vi "fetch_image.vi"(8 "error in (no error)":errorcluster, 11 "GenericToplevelComponent in":refnum<class "GenericToplevelComponent.lvclass">) -> (0 "error out":errorcluster, 1 "channels array empty?":bool, 2 "image (channels)":refnum<class "Image.lvclass">[](array[class]), 3 "GenericToplevelComponent out":refnum<class "GenericToplevelComponent.lvclass">, 4 "# elements in queue":i32, 6 "finished?":bool[](array[boolean]))   [LabVIEW 2010, in "GenericToplevelComponent.lvclass"]
uses:
  GenericToplevelComponent.lvclass
  Image/Image/Image.lvclass
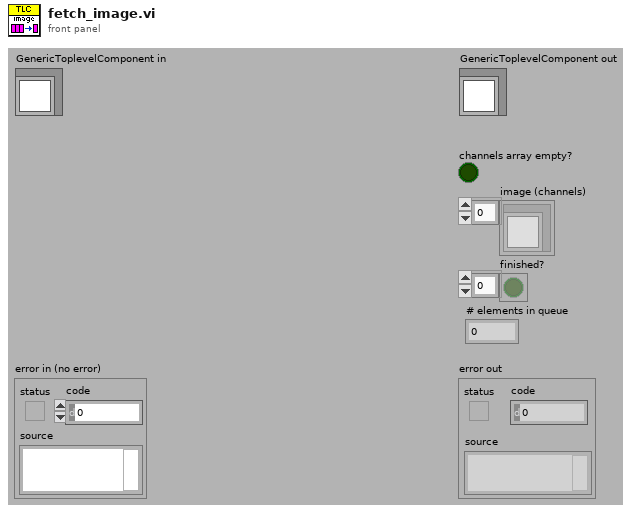
[diagram p1: front panel]
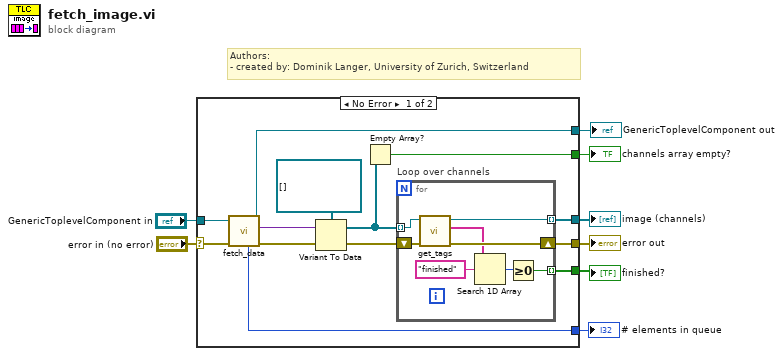
[diagram p0: block diagram]
diagram:
  # "Authors: \n- created by: Dominik Langer, University of Zurich, Switzerland"
  n1 = case shown="No Error" "error in (no error)" {
    selector: "error in (no error)" -> [w18 w31]
    tunnel: [w12 w31] -> w7
    tunnel: [w16 w30] -> w5
    tunnel: "GenericToplevelComponent in" -> [w17 w30]
    tunnel: [w13 _] -> w4
    tunnel: [w11 _] -> w3
    tunnel: [w10 _] -> w2
    tunnel: [w9 _] -> w1
    frame No Error {
      n2 = call-dynamic "fetch_data.vi"("error in (no error)"=w18, "GenericToplevelComponent in"=w17) -> ("error out"=w21:errorcluster, "data out"=w20:variant, "GenericToplevelComponent out"=w16:refnum<class "GenericToplevelComponent.lvclass">, "# elements in queue"=w9:i32)  [unwired: 6 in]
      n3 = Variant To Data(error in=w21, Variant=w20, type=refnum<class "Image.lvclass">[] []) -> (error out=w15:errorcluster, data=w14:refnum<class "Image.lvclass">[])
      n4 = Empty Array?(array=w14) -> (empty?=w13:bool)
      n5 = for "Loop over channels" {
        tunnel: w14 -> [w28] mode=indexing
        shift-right: [w27] -> w12
        shift-left: w15 -> [w29]
        tunnel: [w26] -> w11 mode=indexing
        tunnel: [w22] -> w10 mode=indexing
        n6 = call "get_tags.vi"("error in (no error)"=w29, "Image.lvclass in"=w28) -> ("error out"=w27:errorcluster, "tags"=w25:string[], "Image.lvclass out"=w26:refnum<class "Image.lvclass">)  [unwired: 7 in]
        n7 = Search 1D Array(1D array=w25, element="finished") -> (index of element=w23:i32)  [unwired: 1 in]
        n8 = Greater Or Equal To 0?(x=w23) -> (x >= 0?=w22:bool)
      }
    }
    frame Error {
    }
  }
  "error out" <- w7
  "GenericToplevelComponent out" <- w5
  "channels array empty?" <- w4
  "image (channels)" <- w3
  "finished?" <- w2
  "# elements in queue" <- w1
